vi "group Sync Read.vi"(7 "data_length":u16, 9 "start_address":u16, 10 "protocol_version":i32, 11 "port_num":i32) -> (3 "function return":i32)   [LabVIEW 2016, in "dxl_x86_c.lvlib"]
doc: "WINDECLSPEC int groupSyncRead (int port_num, int protocol_version, uint16_t start_address, uint16_t data_length);"
uses:
  dxl_x86_c.lvlib
  dxl_x86_c.dll
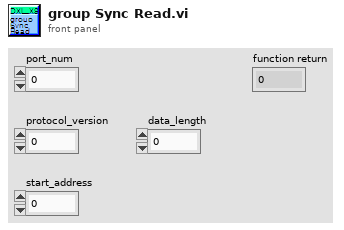
[diagram p1: front panel]
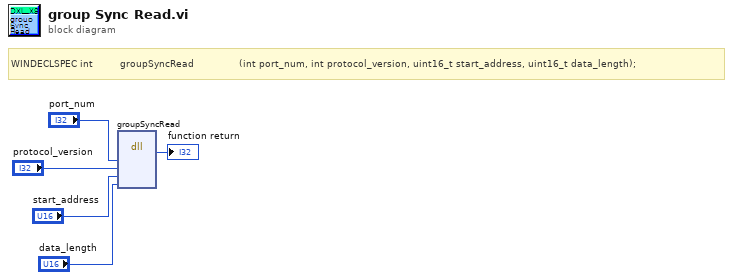
[diagram p0: block diagram]
diagram:
  # "WINDECLSPEC int         groupSyncRead               (int port_num, int protocol_version, uint16_t start_address, uint16_t data_length);"
  n1 = dll-call lib="C:/Users/Platform/Desktop/GITHUB/DynamixelSDK/labview/dxl_x86_c.lvlib/dxl_x86_c.*" fn="groupSyncRead"("port_num"="port_num", "protocol_version"="protocol_version", "start_address"="start_address", "data_length"="data_length") -> (→"function return":i32)  [unwired: 7 in, 2 out]
